vi "Get Node Hierarchy Data RecursiveChild.vi"(9 "Node Hierarchy Data (parent, child)":T1[](array[typedef]), 10 "Node Path (parent, child)":string[](array[string]), 11 "Tree Map In":T3) -> (0 "error out":errorcluster, 1 "Node Hierarchy Data (parent, child)":T1[](array[typedef]), 2 "Node Exists?":bool, 3 "Tree Map Out":T3)   [LabVIEW 2020, in "Blue Tree Map OpenSource.lvlib"]
uses:
  Blue Tree Map OpenSource.lvlib
  Typedefs/Tree Map.ctl
  Typedefs/Tree Map Data.ctl
  Typedefs/Tree Node Data.ctl
  Typedefs/Attribute Map.ctl
  <vilib>/Utility/miscctls.llb/LVMapReplaceAction.ctl
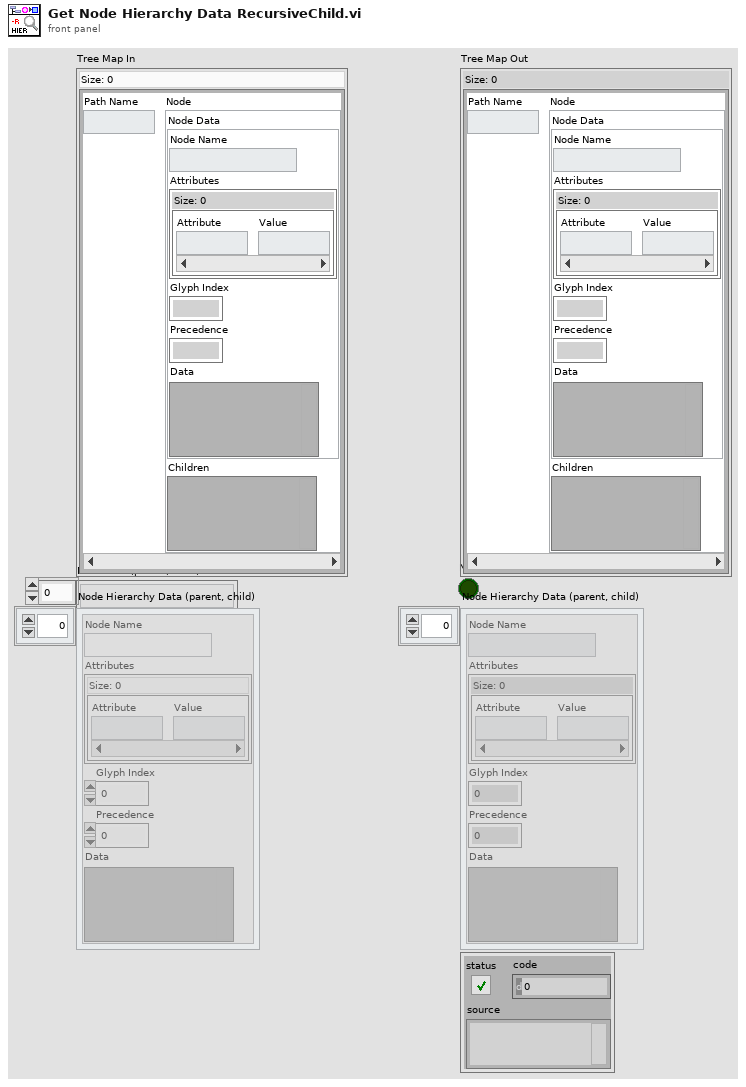
[diagram p1: front panel]
types:
  T1 = typedef "Blue Tree Map OpenSource.lvlib/Tree Node Data.ctl" = cluster{"Node Name":string, "Attributes":T2, "Glyph Index":i32, "Precedence":i32, "Data":variant}
  T2 = typedef "Blue Tree Map OpenSource.lvlib/Attribute Map.ctl" = map{string, string}
  T3 = typedef "Blue Tree Map OpenSource.lvlib/Tree Map.ctl" = map{string, T4}
  T4 = typedef "Blue Tree Map OpenSource.lvlib/Tree Map Data.ctl" = cluster{"Node Data":T1, "Children":variant}
  T5 = typedef "LVMapReplaceAction.ctl" = enum32{"Modify Entry only if found", "Add or Modify Entry", "Delete Entry"}
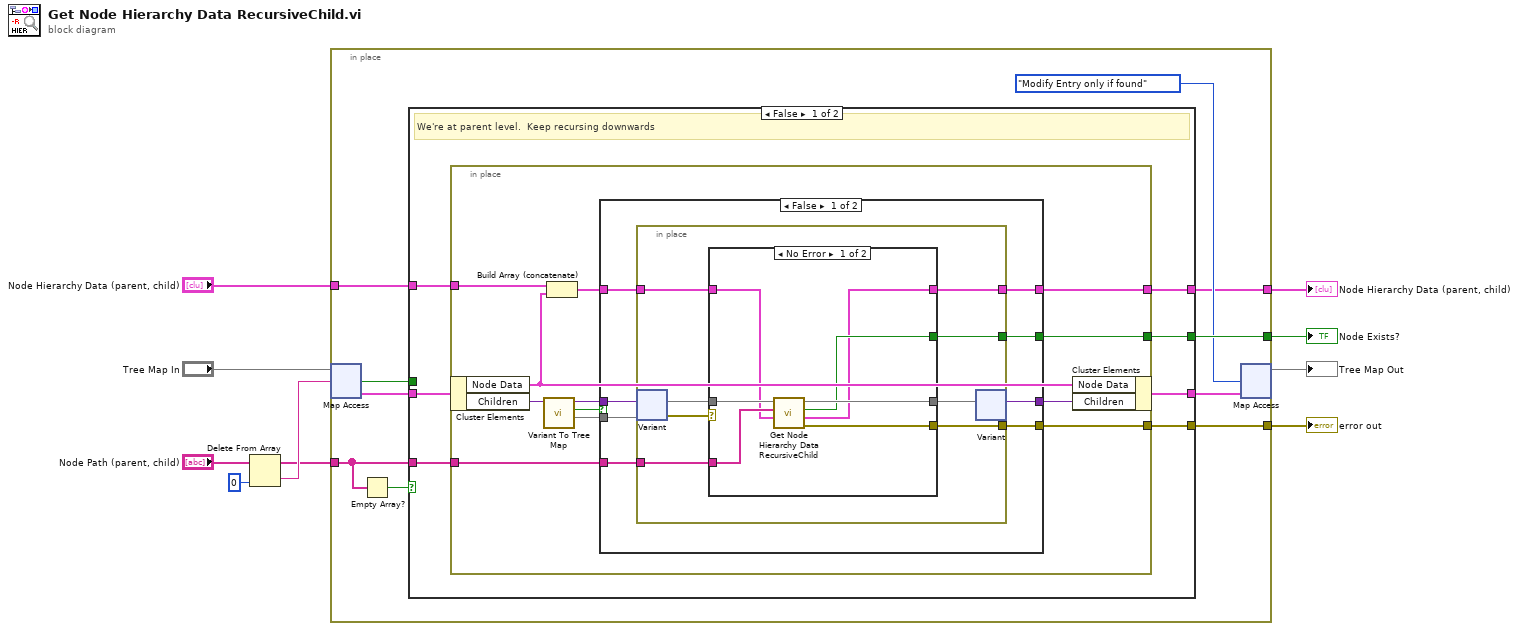
[diagram p0: block diagram]
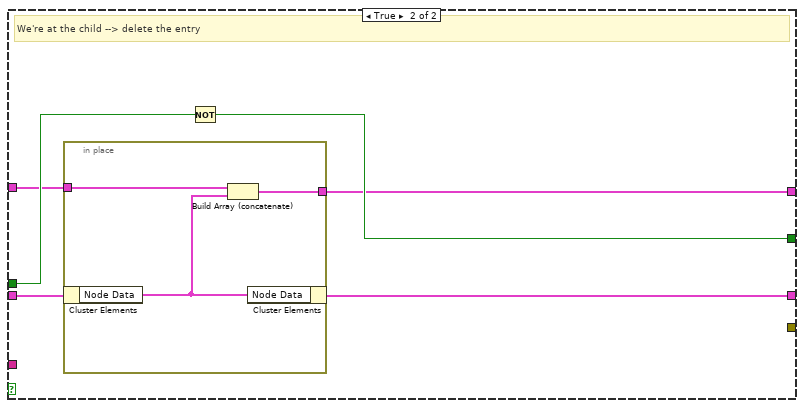
[diagram p4: hidden frame]
diagram:
  n1 = Delete From Array(array="Node Path (parent, child)", index=0) -> (deleted portion=w9:string, array with subset deleted=w8:string[])  [unwired: 1 in]
  n2 = in-place {
    in-place-border: w8 -> [w14]
    in-place-border: [w19] -> w5
    in-place-border: [w17] -> w3
    in-place-border: [w12] -> w1
    in-place-border: "Node Hierarchy Data (parent, child)" -> [w11]
    n3 = in-place-map #1("Tree Map In", w9) -> (w20:T4, w16:bool)  [unwired: 1 in]
    n4 = Empty Array?(array=w14) -> (empty?=w15:bool)
    n5 = case shown="False" w15 {
      tunnel: w20 -> [w27 w71]
      tunnel: w14 -> [w26 _]
      tunnel: [w25 _] -> w19
      tunnel: [w24 w70] -> w18
      tunnel: [w23 w73] -> w17
      tunnel: w16 -> [_ w72]
      tunnel: [w22 w69] -> w12
      tunnel: w11 -> [w21 w68]
      frame False {
        # "We're at parent level.  Keep recursing downwards"
        n6 = in-place {
          in-place-border: w26 -> [w38]
          in-place-border: [w37] -> w25
          in-place-border: [w36] -> w23
          in-place-border: [w31] -> w22
          in-place-border: w21 -> [w30]
          n7 = in-place-cluster #2(w27) -> ("Node Data"=w28:T1, "Children"=w39:variant)
          n8 = call "Variant To Tree Map.vi"("Children"=w39) -> ("Tree Map (Empty)"=w34:T3, "Empty?"=w33:bool, "Children"=w35:variant)  [unwired: 8 in]
          n9 = Build Array (concatenate)(w30, w28) -> (w29:T1[])
          n10 = case shown="False" w33 {
            tunnel: w38 -> [w47 _]
            tunnel: [w46 _] -> w37
            tunnel: [w45 _] -> w36
            tunnel: w35 -> [w44 w67]
            tunnel: w34 -> [w43 _]
            tunnel: [w42 w67] -> w32
            tunnel: [w41 w66] -> w31
            tunnel: w29 -> [w40 w66]
            frame False {
              n11 = in-place {
                in-place-border: w47 -> [w55]
                in-place-border: [w54] -> w46
                in-place-border: [w53] -> w45
                in-place-border: [w49] -> w41
                in-place-border: w40 -> [w48]
                n12 = in-place-variant #3(w44, w43) -> (w52:T3, w50:errorcluster)
                n13 = case shown="No Error" w50 {
                  selector: w50 -> [_ w64]
                  tunnel: w55 -> [w59 _]
                  tunnel: [w60 w64] -> w54
                  tunnel: [w58 _] -> w53
                  tunnel: w52 -> [w62 w65]
                  tunnel: [w61 w65] -> w51
                  tunnel: [w56 w63] -> w49
                  tunnel: w48 -> [w57 w63]
                  frame No Error {
                    n14 = call "Get Node Hierarchy Data RecursiveChild.vi"("Node Hierarchy Data (parent, child)"=w57, "Node Path (parent, child)"=w59, "Tree Map In"=w62) -> ("error out"=w60:errorcluster, "Node Hierarchy Data (parent, child)"=w56:T1[], "Node Exists?"=w58:bool, "Tree Map Out"=w61:T3)  [unwired: 5 in]
                  }
                  frame Error {
                  }
                }
                n15 = in-place-variant #3(w51) -> (w42:variant)  [unwired: 1 out]
              }
            }
            frame True {
            }
          }
          n16 = in-place-cluster #2("Node Data"=w28, "Children"=w32) -> (w24:T4)
        }
      }
      frame True {
        # "We're at the child --> delete the entry"
        n17 = in-place {
          in-place-border: [w76] -> w69
          in-place-border: w68 -> [w74]
          n18 = in-place-cluster #4(w71) -> ("Node Data"=w75:T1)
          n19 = Build Array (concatenate)(w74, w75) -> (w76:T1[])
          n20 = in-place-cluster #4("Node Data"=w75) -> (w70:T4)
        }
        n21 = Not(x=w72) -> (.not. x?=w73:bool)
      }
    }
    n22 = in-place-map #1(w18, LVMapReplaceAction."Modify Entry only if found" ("action")) -> (→"Tree Map Out":T3)  [unwired: 2 out]
  }
  "error out" <- w5
  "Node Exists?" <- w3
  "Node Hierarchy Data (parent, child)" <- w1
